vi "Get flattened data.vi"(8 "error in (no error)":errorcluster, 11 "Float D Element in":refnum<class "Float D Element.lvclass">) -> (0 "error out":errorcluster, 2 "Flattened data":u8[](array[numeric]), 3 "Float D Element out":refnum<class "Float D Element.lvclass">)   [LabVIEW 2018, in "D Datagrid Library.lvlib" / "Float D Element.lvclass"]
uses:
  Float D Element.lvclass
  Float D Element.lvclass/Float D Element.ctl
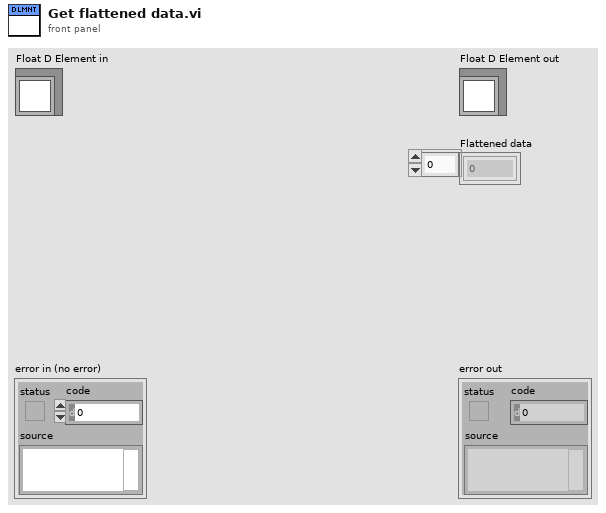
[diagram p1: front panel]
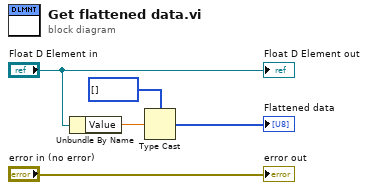
[diagram p0: block diagram]
diagram:
  n1 = Unbundle By Name("Float D Element in") -> ("Value"=w3:sgl)
  n2 = Type Cast(type=u8[] [] ("Flattened data"), x=w3) -> (*(type *) &x=→"Flattened data":u8[])
  "error out" <- "error in (no error)"
  "Float D Element out" <- "Float D Element in"
